vi "INSTRUMENTORDERS.vi"(0 "VISA资源名称":refnum<visa-resource-name>="DPO5054-C012667", 1 "打开通道":u16(ring) items=["CH1", "CH2", "CH3", "CH4"], 2 "关闭通道":u16(ring) items=["CH1", "CH2", "CH3", "CH4"], 5 "错误输入（无错误）":errorcluster) -> (11 "FREQ":dbl, 12 "VISA资源名称输出":refnum<visa-resource-name>, 13 "PERIOD":dbl, 14 "RMS":dbl, 15 "AMP":dbl, 16 "MAX":dbl, 17 "MIN":dbl, 18 "PK2PK":dbl, 19 "错误输出":errorcluster)   [LabVIEW 2014]
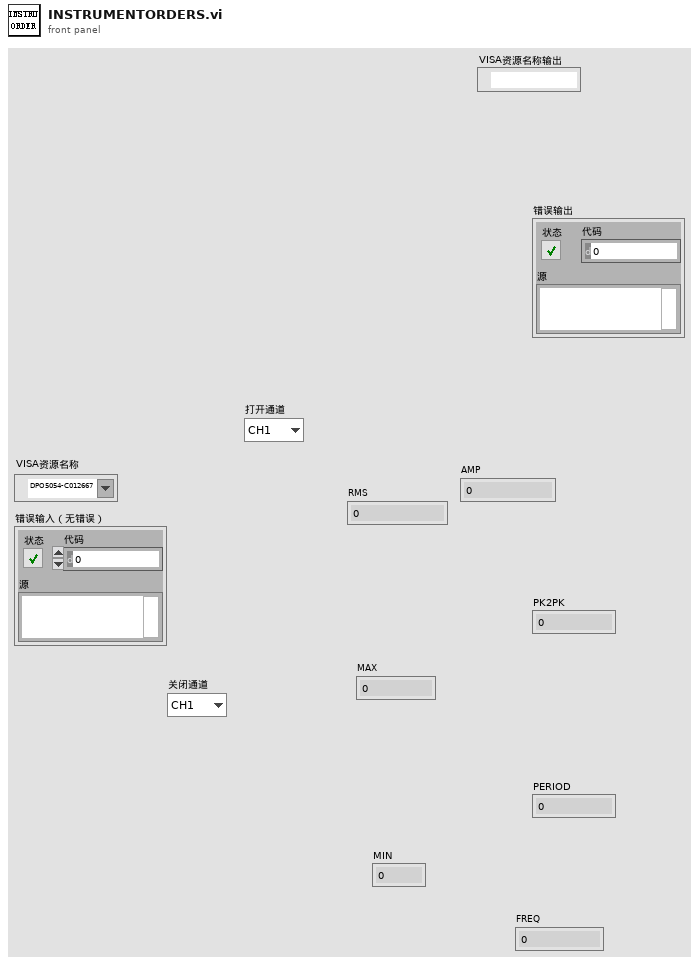
[diagram p1: front panel]
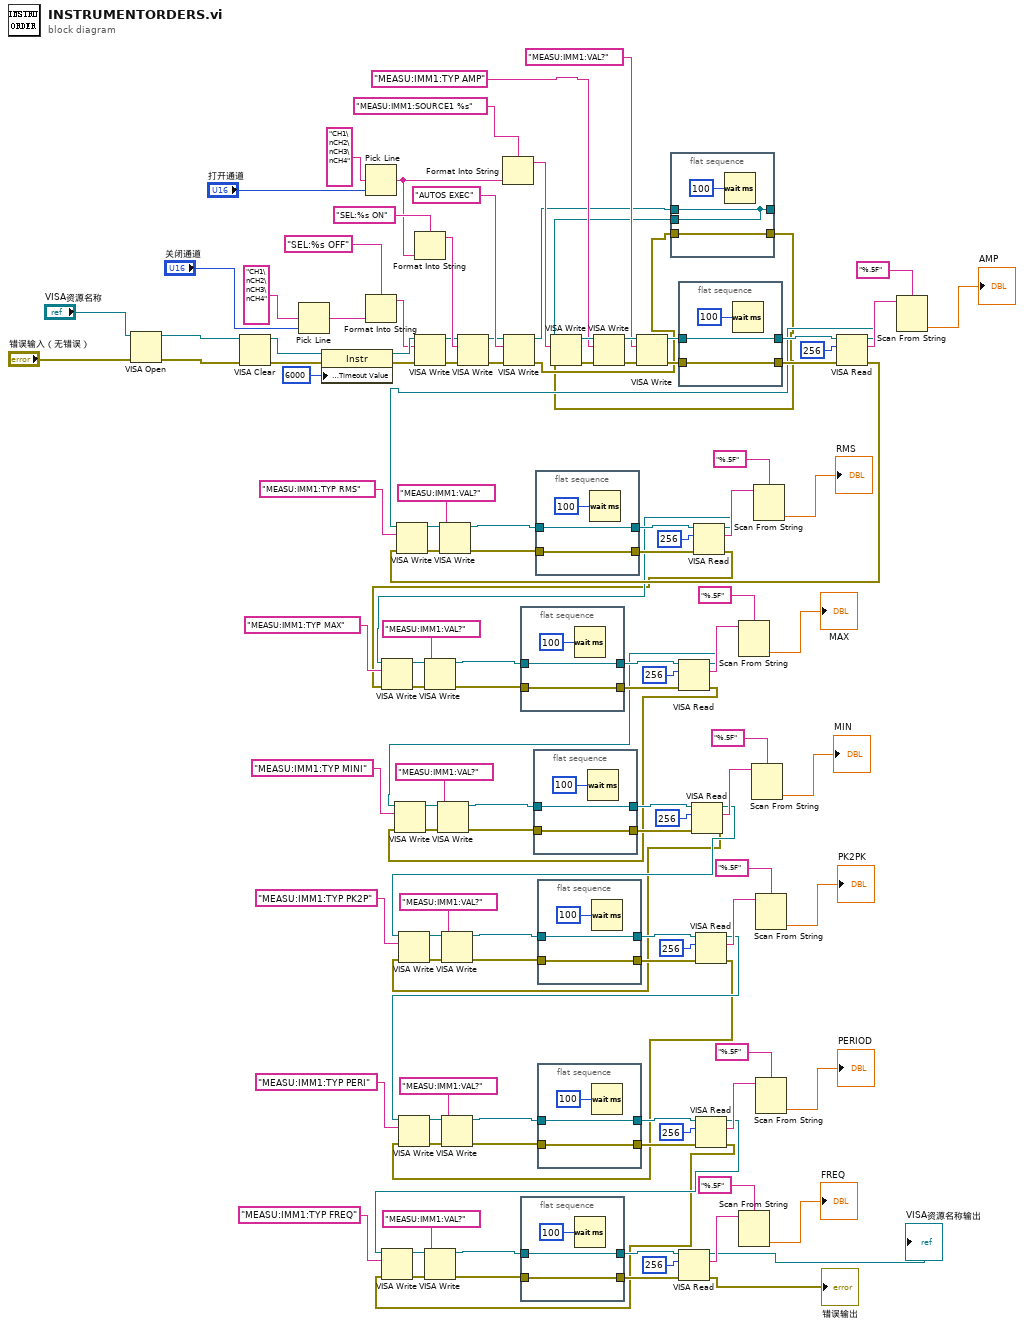
[diagram p0: block diagram]
diagram:
  n1 = VISA Open(error in (no error)="错误输入（无错误）", VISA resource name="VISA资源名称") -> (VISA resource name=w129:refnum<visa-resource-name>, error out=w128:errorcluster)  [unwired: 3 in]
  n2 = VISA Clear(VISA resource name=w129, error in (no error)=w128) -> (VISA resource name out=w127:refnum<visa-resource-name>, error out=w126:errorcluster)
  n3 = Pick Line(multi-line string="CH1\nCH2\nCH3\nCH4" ("多行字符串"), line index="关闭通道") -> (output string=w101:string)  [unwired: 1 in]
  n4 = property class="Instr"(reference=w127, error in=w126, "General Settings:Timeout Value"=u32 6000) -> (reference out=w103:refnum<visa-resource-name>, error out=w102:errorcluster)
  n5 = Pick Line(multi-line string="CH1\nCH2\nCH3\nCH4" ("多行字符串"), line index="打开通道") -> (output string=w108:string)  [unwired: 1 in]
  n6 = Format Into String(format string="SEL:%s OFF" ("格式字符串"), w101) -> (resulting string=w97:string)  [unwired: 2 in, 1 out]
  n7 = Format Into String(format string="SEL:%s ON" ("格式字符串"), w108) -> (resulting string=w107:string)  [unwired: 2 in, 1 out]
  n8 = VISA Write(VISA resource name=w103, write buffer=w97, error in (no error)=w102) -> (VISA resource name out=w96:refnum<visa-resource-name>, error out=w95:errorcluster)  [unwired: 1 out]
  n9 = VISA Write(VISA resource name=w96, write buffer=w107, error in (no error)=w95) -> (VISA resource name out=w105:refnum<visa-resource-name>, error out=w104:errorcluster)  [unwired: 1 out]
  n10 = Format Into String(format string="MEASU:IMM1:SOURCE1 %s" ("格式字符串"), w108) -> (resulting string=w121:string)  [unwired: 2 in, 1 out]
  n11 = VISA Write(VISA resource name=w105, write buffer="AUTOS EXEC" ("写入缓冲区"), error in (no error)=w104) -> (VISA resource name out=w5:refnum<visa-resource-name>, error out=w4:errorcluster)  [unwired: 1 out]
  n12 = flat-sequence {
    tunnel: w77 -> [w132]
    tunnel: [w132] -> w75
    tunnel: w78 -> [w131]
    tunnel: [w131] -> w74
    frame #0 {
      n13 = Wait (ms)(milliseconds to wait=u32 100 ("等待时间（毫秒）")) -> ()  [unwired: 1 out]
    }
  }
  n14 = flat-sequence {
    tunnel: w29 -> [w135]
    tunnel: [w135] -> w27
    tunnel: w30 -> [w134]
    tunnel: [w134] -> w26
    frame #0 {
      n15 = Wait (ms)(milliseconds to wait=u32 100 ("等待时间（毫秒）")) -> ()  [unwired: 1 out]
    }
  }
  n16 = flat-sequence {
    tunnel: w56 -> [w138]
    tunnel: [w138] -> w58
    tunnel: w55 -> [w137]
    tunnel: [w137] -> w59
    frame #0 {
      n17 = Wait (ms)(milliseconds to wait=u32 100 ("等待时间（毫秒）")) -> ()  [unwired: 1 out]
    }
  }
  n18 = flat-sequence {
    tunnel: w80 -> [w141]
    tunnel: [w141] -> w82
    tunnel: w79 -> [w140]
    tunnel: [w140] -> w83
    frame #0 {
      n19 = Wait (ms)(milliseconds to wait=u32 100 ("等待时间（毫秒）")) -> ()  [unwired: 1 out]
    }
  }
  n20 = flat-sequence {
    tunnel: w53 -> [w144]
    tunnel: [w144] -> w51
    tunnel: w54 -> [w143]
    tunnel: [w143] -> w50
    frame #0 {
      n21 = Wait (ms)(milliseconds to wait=u32 100 ("等待时间（毫秒）")) -> ()  [unwired: 1 out]
    }
  }
  n22 = flat-sequence {
    tunnel: w32 -> [w147]
    tunnel: [w147] -> w34
    tunnel: w31 -> [w146]
    tunnel: [w146] -> w35
    frame #0 {
      n23 = Wait (ms)(milliseconds to wait=u32 100 ("等待时间（毫秒）")) -> ()  [unwired: 1 out]
    }
  }
  n24 = VISA Write(VISA resource name=w3, write buffer=w121, error in (no error)=w2) -> (VISA resource name out=w118:refnum<visa-resource-name>, error out=w117:errorcluster)  [unwired: 1 out]
  n25 = VISA Write(VISA resource name=w118, write buffer="MEASU:IMM1:TYP AMP" ("写入缓冲区"), error in (no error)=w117) -> (VISA resource name out=w114:refnum<visa-resource-name>, error out=w113:errorcluster)  [unwired: 1 out]
  n26 = VISA Write(VISA resource name=w114, write buffer="MEASU:IMM1:VAL?" ("写入缓冲区"), error in (no error)=w113) -> (VISA resource name out=w111:refnum<visa-resource-name>, error out=w110:errorcluster)  [unwired: 1 out]
  n27 = flat-sequence {
    tunnel: w5 -> [w149]
    tunnel: [w149] -> _
    tunnel: w4 -> [w150]
    tunnel: [w150] -> w2
    tunnel: [w149] -> w3
    frame #0 {
      n28 = Wait (ms)(milliseconds to wait=u32 100 ("等待时间（毫秒）")) -> ()  [unwired: 1 out]
    }
  }
  n29 = flat-sequence {
    tunnel: w111 -> [w153]
    tunnel: [w153] -> w116
    tunnel: w110 -> [w152]
    tunnel: [w152] -> w115
    frame #0 {
      n30 = Wait (ms)(milliseconds to wait=u32 100 ("等待时间（毫秒）")) -> ()  [unwired: 1 out]
    }
  }
  n31 = VISA Read(VISA resource name=w75, byte count=u32 256 ("字节总数"), error in (no error)=w74) -> (VISA resource name out=w14:refnum<visa-resource-name>, read buffer=w73:string, error out=w13:errorcluster)  [unwired: 1 out]
  n32 = VISA Write(VISA resource name=w14, write buffer="MEASU:IMM1:TYP MINI" ("写入缓冲区"), error in (no error)=w13) -> (VISA resource name out=w64:refnum<visa-resource-name>, error out=w65:errorcluster)  [unwired: 1 out]
  n33 = VISA Write(VISA resource name=w64, write buffer="MEASU:IMM1:VAL?" ("写入缓冲区"), error in (no error)=w65) -> (VISA resource name out=w56:refnum<visa-resource-name>, error out=w55:errorcluster)  [unwired: 1 out]
  n34 = VISA Read(VISA resource name=w27, byte count=u32 256 ("字节总数"), error in (no error)=w26) -> (VISA resource name out=→"VISA资源名称输出":refnum<visa-resource-name>, read buffer=w25:string, error out=→"错误输出":errorcluster)  [unwired: 1 out]
  n35 = VISA Read(VISA resource name=w58, byte count=u32 256 ("字节总数"), error in (no error)=w59) -> (VISA resource name out=w12:refnum<visa-resource-name>, read buffer=w60:string, error out=w11:errorcluster)  [unwired: 1 out]
  n36 = VISA Write(VISA resource name=w12, write buffer="MEASU:IMM1:TYP PK2P" ("写入缓冲区"), error in (no error)=w11) -> (VISA resource name out=w45:refnum<visa-resource-name>, error out=w44:errorcluster)  [unwired: 1 out]
  n37 = VISA Write(VISA resource name=w45, write buffer="MEASU:IMM1:VAL?" ("写入缓冲区"), error in (no error)=w44) -> (VISA resource name out=w53:refnum<visa-resource-name>, error out=w54:errorcluster)  [unwired: 1 out]
  n38 = VISA Read(VISA resource name=w82, byte count=u32 256 ("字节总数"), error in (no error)=w83) -> (VISA resource name out=w16:refnum<visa-resource-name>, read buffer=w84:string, error out=w15:errorcluster)  [unwired: 1 out]
  n39 = VISA Write(VISA resource name=w16, write buffer="MEASU:IMM1:TYP MAX" ("写入缓冲区"), error in (no error)=w15) -> (VISA resource name out=w69:refnum<visa-resource-name>, error out=w68:errorcluster)  [unwired: 1 out]
  n40 = VISA Write(VISA resource name=w69, write buffer="MEASU:IMM1:VAL?" ("写入缓冲区"), error in (no error)=w68) -> (VISA resource name out=w77:refnum<visa-resource-name>, error out=w78:errorcluster)  [unwired: 1 out]
  n41 = VISA Read(VISA resource name=w51, byte count=u32 256 ("字节总数"), error in (no error)=w50) -> (VISA resource name out=w10:refnum<visa-resource-name>, read buffer=w49:string, error out=w9:errorcluster)  [unwired: 1 out]
  n42 = VISA Write(VISA resource name=w10, write buffer="MEASU:IMM1:TYP PERI" ("写入缓冲区"), error in (no error)=w9) -> (VISA resource name out=w40:refnum<visa-resource-name>, error out=w41:errorcluster)  [unwired: 1 out]
  n43 = VISA Write(VISA resource name=w40, write buffer="MEASU:IMM1:VAL?" ("写入缓冲区"), error in (no error)=w41) -> (VISA resource name out=w32:refnum<visa-resource-name>, error out=w31:errorcluster)  [unwired: 1 out]
  n44 = VISA Read(VISA resource name=w34, byte count=u32 256 ("字节总数"), error in (no error)=w35) -> (VISA resource name out=w8:refnum<visa-resource-name>, read buffer=w36:string, error out=w7:errorcluster)  [unwired: 1 out]
  n45 = VISA Write(VISA resource name=w8, write buffer="MEASU:IMM1:TYP FREQ" ("写入缓冲区"), error in (no error)=w7) -> (VISA resource name out=w21:refnum<visa-resource-name>, error out=w20:errorcluster)  [unwired: 1 out]
  n46 = VISA Write(VISA resource name=w21, write buffer="MEASU:IMM1:VAL?" ("写入缓冲区"), error in (no error)=w20) -> (VISA resource name out=w29:refnum<visa-resource-name>, error out=w30:errorcluster)  [unwired: 1 out]
  n47 = Scan From String(format string="%.5F" ("格式字符串"), input string=w73) -> (output 1=→"MAX":dbl)  [unwired: 3 in, 3 out]
  n48 = Scan From String(format string="%.5F" ("格式字符串"), input string=w25) -> (output 1=→"FREQ":dbl)  [unwired: 3 in, 3 out]
  n49 = Scan From String(format string="%.5F" ("格式字符串"), input string=w60) -> (output 1=→"MIN":dbl)  [unwired: 3 in, 3 out]
  n50 = Scan From String(format string="%.5F" ("格式字符串"), input string=w84) -> (output 1=→"RMS":dbl)  [unwired: 3 in, 3 out]
  n51 = Scan From String(format string="%.5F" ("格式字符串"), input string=w49) -> (output 1=→"PK2PK":dbl)  [unwired: 3 in, 3 out]
  n52 = Scan From String(format string="%.5F" ("格式字符串"), input string=w36) -> (output 1=→"PERIOD":dbl)  [unwired: 3 in, 3 out]
  n53 = VISA Read(VISA resource name=w116, byte count=u32 256 ("字节总数"), error in (no error)=w115) -> (VISA resource name out=w18:refnum<visa-resource-name>, read buffer=w93:string, error out=w17:errorcluster)  [unwired: 1 out]
  n54 = VISA Write(VISA resource name=w18, write buffer="MEASU:IMM1:TYP RMS" ("写入缓冲区"), error in (no error)=w17) -> (VISA resource name out=w88:refnum<visa-resource-name>, error out=w89:errorcluster)  [unwired: 1 out]
  n55 = VISA Write(VISA resource name=w88, write buffer="MEASU:IMM1:VAL?" ("写入缓冲区"), error in (no error)=w89) -> (VISA resource name out=w80:refnum<visa-resource-name>, error out=w79:errorcluster)  [unwired: 1 out]
  n56 = Scan From String(format string="%.5F" ("格式字符串"), input string=w93) -> (output 1=→"AMP":dbl)  [unwired: 3 in, 3 out]
